vi "(SubVI)Launcher_HTTP Simple Status Code Handler.vi"(0 "client handle in":T1 caption="클라이언트 핸들 출력", 5 "HTTP Header":string, 11 "error in (no error)":errorcluster caption="에러 입력(에러 없음)") -> (4 "client handle out":T1 caption="클라이언트 핸들 출력", 6 "Header":string, 8 "Success?":bool, 10 "Status Code":dbl, 14 "Message":string, 15 "error out":errorcluster caption="에러 출력")   [LabVIEW 2020]
uses:
  <vilib>/httpClient/ClientHandle.ctl
  <vilib>/httpClient/LabVIEWHTTPClient.lvlib
panel:
  out "HTTP Version":dbl
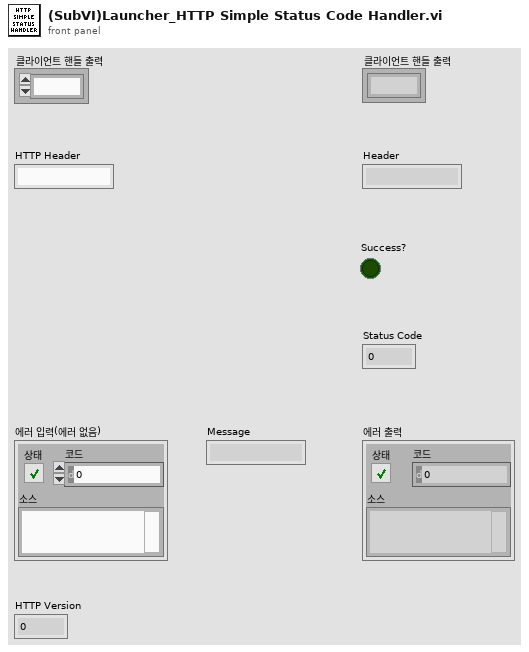
[diagram p1: front panel]
types:
  T1 = typedef "LabVIEWHTTPClient.lvlib/ClientHandle.ctl" = refnum<k1>
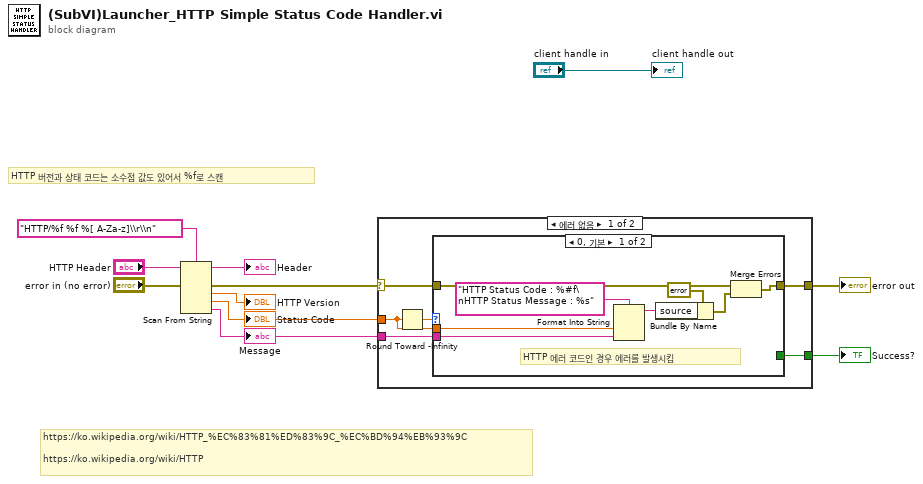
[diagram p0: block diagram]
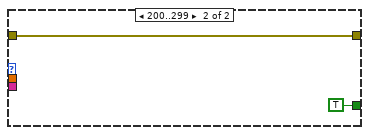
[diagram p2: hidden frame]
diagram:
  # "HTTP 버전과 상태 코드는 소수점 값도 있어서 %f로 스캔"
  # "https://ko.wikipedia.org/wiki/HTTP_%EC%83%81%ED%83%9C_%EC%BD%94%EB%93%9C\n\nhttps://ko.wikipedia.org/wiki/HTTP"
  n1 = Scan From String(format string="HTTP/%f %f %[ A-Za-z]\\r\\n" ("포맷 문자열"), input string="HTTP Header", error in="error in (no error)") -> (remaining string=→"Header":string, error out=w6:errorcluster, output 1=→"HTTP Version":dbl, output 2=w5:dbl, output 3=w3:string)  [unwired: 4 in, 1 out]
  "Status Code" <- w5
  "Message" <- w3
  n2 = case shown="에러 없음" w6 {
    selector: w6 -> [w17 w28]
    tunnel: [w16 w28] -> w4
    tunnel: w5 -> [w14 _]
    tunnel: w3 -> [w13 _]
    tunnel: [w12 _] -> w1
    frame No Error {
      n3 = Round Toward -Infinity(1:w14) -> (0:w15:dbl)
      n4 = case shown="0, 기본" w15 {
        tunnel: w17 -> [w25 w27]
        tunnel: [w24 w27] -> w16
        tunnel: w14 -> [w22 _]
        tunnel: w13 -> [w18 _]
        tunnel: [_ TRUE] -> w12
        frame 0, Default {
          # "HTTP 에러 코드인 경우 에러를 발생시킴"
          n5 = Format Into String(format string="HTTP Status Code : %#f\nHTTP Status Message : %s" ("포맷 문자열"), w22, w18) -> (resulting string=w20:string)  [unwired: 2 in, 1 out]
          n6 = Bundle By Name(cluster=errorcluster {"status"=TRUE, "code"=0, "source"=""} ("에러 입력"), "source"=w20) -> (w19:errorcluster)
          n7 = Merge Errors(w25, w19) -> (w24:errorcluster)
        }
        frame 200..299 {
        }
      }
    }
    frame Error {
    }
  }
  "error out" <- w4
  "Success?" <- w1
  "client handle out" <- "client handle in"
